vi "calculatefit.vi"(11 "input":dbl[][](array[numeric])) -> (3 "output":dbl[](array[numeric]))   [LabVIEW 2012]
uses:
  <vilib>/Analysis/NI_AALPro.lvlib
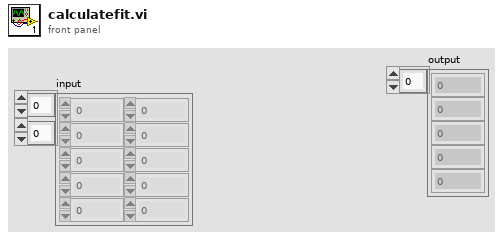
[diagram p1: front panel]
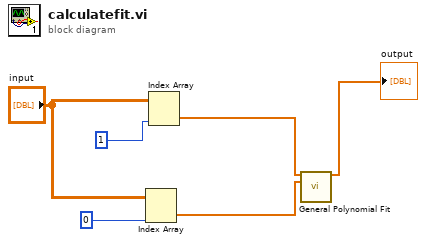
[diagram p0: block diagram]
diagram:
  n1 = Index Array(array="input", index (col)=0) -> (element=w2:dbl[])  [unwired: 1 in]
  n2 = Index Array(array="input", index (col)=1) -> (element=w3:dbl[])  [unwired: 1 in]
  n3 = call <vilib>:"General Polynomial Fit.vi"("Y"=w3, "X"=w2) -> ("Best Polynomial Fit"=→"output":dbl[])  [unwired: 10 in, 3 out]
